vi "Read File.vi"(8 "error in (no error)":errorcluster, 10 "Parameters":refnum<class "Parameter.lvclass">[](array[class]), 11 "Parameter INI File in":refnum<class "Parameter INI File.lvclass">) -> (0 "error out":errorcluster, 2 "Parameters":refnum<class "Parameter.lvclass">[](array[class]), 3 "Parameter INI File out":refnum<class "Parameter INI File.lvclass">)   [LabVIEW 2016, in "CD Parameter Manager API.lvlib" / "Parameter INI File.lvclass"]
uses:
  Parameter INI File.lvclass
  <vilib>/Utility/config.llb/NI_LVConfig.lvlib
  <vilib>/Utility/error.llb/Error Cluster From Error Code.vi
  <vilib>/ErrorRing/Error Ring.xnode
  Boolean Parameter Class/Boolean Parameter.lvclass
  I32 Parameter Class/I32 Parameter.lvclass
  <vilib>/Utility/config.llb/Read Key (Boolean).vi
  <vilib>/Utility/config.llb/Read Key (I32).vi
  Double Parameter Class/Double Parameter.lvclass
  <vilib>/Utility/config.llb/Read Key (Double).vi
  String Parameter Class/String Parameter.lvclass
  <vilib>/Utility/config.llb/Read Key (String).vi
  Parameter Class/Parameter.lvclass
  <vilib>/Utility/config.llb/Read Key (Path).vi
  File Path Parameter Class/File Path Parameter.lvclass
  C:/Repositories/UI-Control-Initializer-API/Source/Parameter Class/Parameter.lvclass
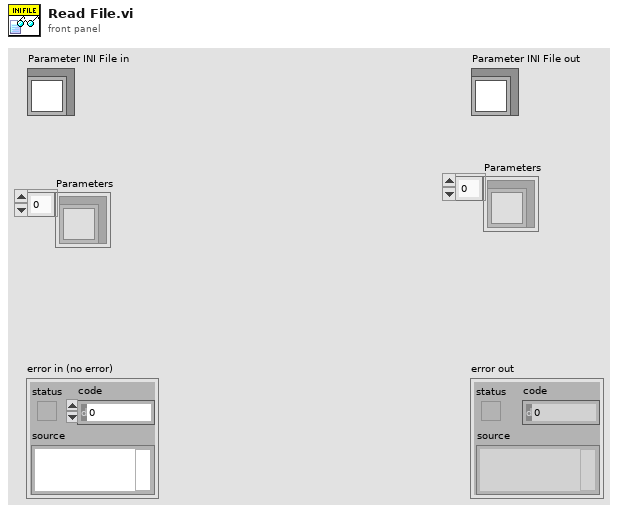
[diagram p1: front panel]
types:
  T1 = typedef "NI_LVConfig.lvlib/Config Data RefNum.ctl" = refnum<k1>
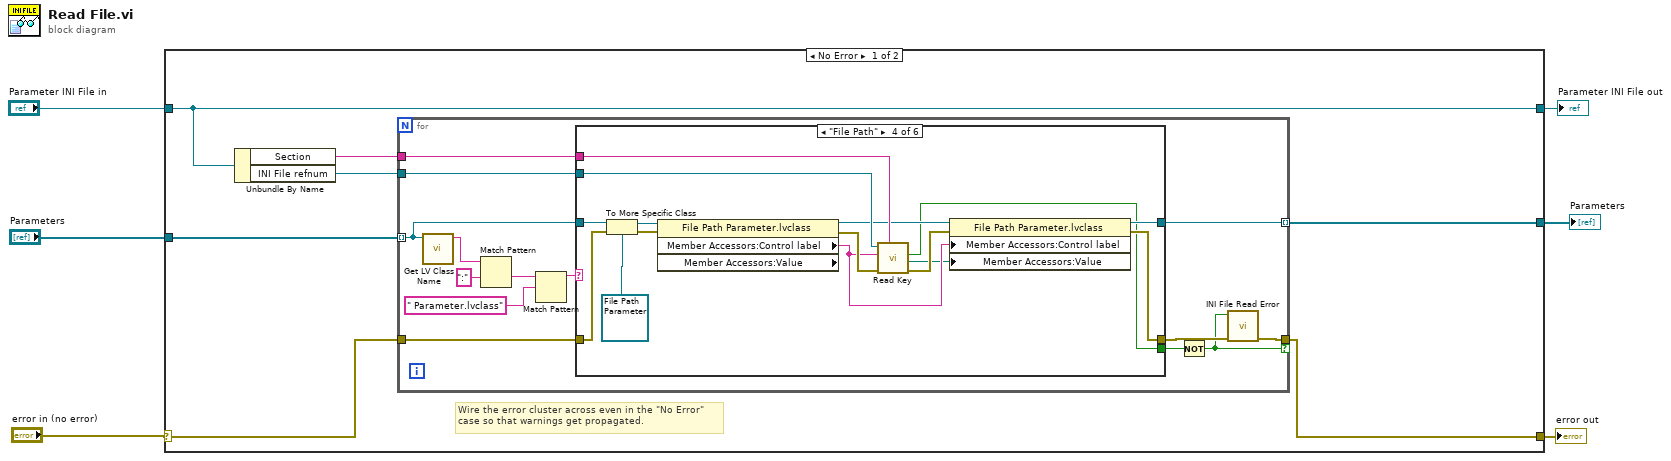
[diagram p0: block diagram]
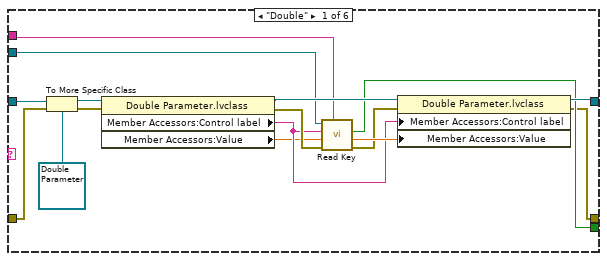
[diagram p2: hidden frame]
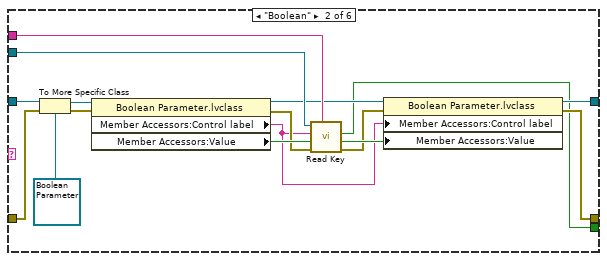
[diagram p3: hidden frame]
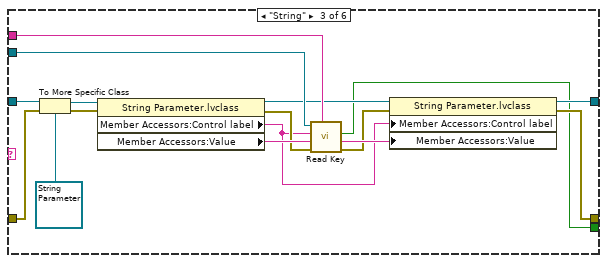
[diagram p4: hidden frame]
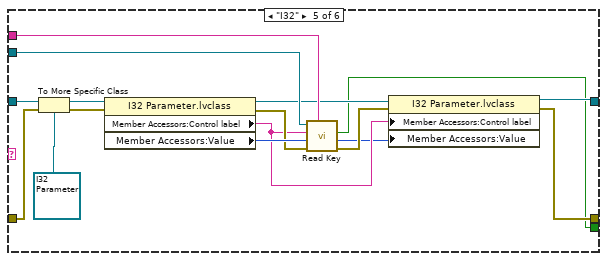
[diagram p5: hidden frame]
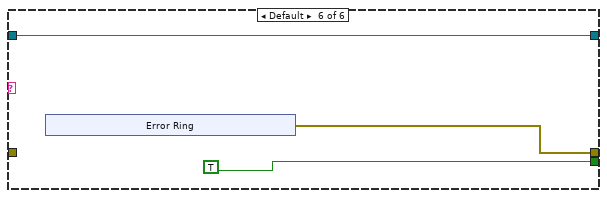
[diagram p6: hidden frame]
diagram:
  n1 = case shown="No Error" "error in (no error)" {
    selector: "error in (no error)" -> [w13 w117]
    tunnel: [w8 w117] -> w4
    tunnel: [w10 w116] -> w5
    tunnel: "Parameter INI File in" -> [w10 w116]
    tunnel: "Parameters" -> [w9 w115]
    tunnel: [w7 w115] -> w1
    frame No Error {
      # "Wire the error cluster across even in the \"No Error\"\ncase so that warnings get propagated."
      n2 = Unbundle By Name(w10) -> ("Section"=w11:string, "INI File refnum"=w12:T1)
      n3 = for {
        tunnel: w13 -> [w22]
        tunnel: [w15] -> w8 if=w14
        tunnel: w12 -> [w20]
        tunnel: w9 -> [w19] mode=indexing
        tunnel: w11 -> [w18]
        tunnel: [w17] -> w7 mode=indexing
        n4 = call <vilib>:"Get LV Class Name.vi"("object"=w19) -> ("class name"=w24:string)  [unwired: 9 in, 1 out]
        n5 = Match Pattern(string=w24, regular expression=":") -> (after substring=w26:string)  [unwired: 1 in, 3 out]
        n6 = Match Pattern(string=w26, regular expression=" Parameter.lvclass") -> (before substring=w23:string)  [unwired: 1 in, 3 out]
        n7 = case shown="\"File Path\"" w23 {
          tunnel: w22 -> [w39 w55 w71 w87 w102 _]
          tunnel: [w30 w46 w63 w80 w93 w108] -> w16
          tunnel: [w31 w44 w61 w78 w91 TRUE] -> w21
          tunnel: w20 -> [w28 w52 w68 w84 w100 _]
          tunnel: w19 -> [w42 w56 w72 w88 w103 w107]
          tunnel: w18 -> [w29 w53 w69 w85 w99 _]
          tunnel: [w32 w45 w62 w79 w96 w107] -> w17
          frame "Double" {
            n8 = To More Specific Class(target class=refnum<class "Double Parameter.lvclass"> refnum ("CD Parameter Manager API.lvlib:Double Parameter.lvclass"), reference=w42, error in=w39) -> (specific class reference=w41:refnum<class "Double Parameter.lvclass">, error out=w43:errorcluster)
            n9 = property class="Double Parameter.lvclass"(reference=w41, error in=w43) -> (reference out=w36:refnum<class "Double Parameter.lvclass">, error out=w35:errorcluster, "Member Accessors:Control label"=w34:string, "Member Accessors:Value"=w33:dbl)
            n10 = call-poly <vilib>:"Read Key.vi"("section"=w29, "error in (no error)"=w35, "default value"=w33, "key"=w34, "refnum"=w28) -> ("error out"=w37:errorcluster, "value"=w38:dbl, "found?"=w31:bool)  [unwired: 3 in, 1 out]
            n11 = property class="Double Parameter.lvclass"(reference=w36, error in=w37, "Member Accessors:Control label"=w34, "Member Accessors:Value"=w38) -> (reference out=w32:refnum<class "Double Parameter.lvclass">, error out=w30:errorcluster)
          }
          frame "Boolean" {
            n12 = To More Specific Class(target class=refnum<class "Boolean Parameter.lvclass"> refnum ("CD Parameter Manager API.lvlib:Boolean Parameter.lvclass"), reference=w56, error in=w55) -> (specific class reference=w58:refnum<class "Boolean Parameter.lvclass">, error out=w59:errorcluster)
            n13 = property class="Boolean Parameter.lvclass"(reference=w58, error in=w59) -> (reference out=w48:refnum<class "Boolean Parameter.lvclass">, error out=w54:errorcluster, "Member Accessors:Control label"=w47:string, "Member Accessors:Value"=w57:bool)
            n14 = call-poly <vilib>:"Read Key.vi"("section"=w53, "error in (no error)"=w54, "default value"=w57, "key"=w47, "refnum"=w52) -> ("error out"=w49:errorcluster, "value"=w50:bool, "found?"=w44:bool)  [unwired: 3 in, 1 out]
            n15 = property class="Boolean Parameter.lvclass"(reference=w48, error in=w49, "Member Accessors:Control label"=w47, "Member Accessors:Value"=w50) -> (reference out=w45:refnum<class "Boolean Parameter.lvclass">, error out=w46:errorcluster)
          }
          frame "String" {
            n16 = To More Specific Class(target class=refnum<class "String Parameter.lvclass"> refnum ("CD Parameter Manager API.lvlib:String Parameter.lvclass"), reference=w72, error in=w71) -> (specific class reference=w74:refnum<class "String Parameter.lvclass">, error out=w75:errorcluster)
            n17 = property class="String Parameter.lvclass"(reference=w74, error in=w75) -> (reference out=w65:refnum<class "String Parameter.lvclass">, error out=w70:errorcluster, "Member Accessors:Control label"=w64:string, "Member Accessors:Value"=w73:string)
            n18 = call-poly <vilib>:"Read Key.vi"("section"=w69, "error in (no error)"=w70, "default value"=w73, "key"=w64, "refnum"=w68) -> ("error out"=w66:errorcluster, "value"=w67:string, "found?"=w61:bool)  [unwired: 3 in, 1 out]
            n19 = property class="String Parameter.lvclass"(reference=w65, error in=w66, "Member Accessors:Control label"=w64, "Member Accessors:Value"=w67) -> (reference out=w62:refnum<class "String Parameter.lvclass">, error out=w63:errorcluster)
          }
          frame "File Path" {
            n20 = To More Specific Class(target class=refnum<class "File Path Parameter.lvclass"> refnum ("CD Parameter Manager API.lvlib:File Path Parameter.lvclass"), reference=w88, error in=w87) -> (specific class reference=w89:refnum<class "File Path Parameter.lvclass">, error out=w90:errorcluster)
            n21 = property class="File Path Parameter.lvclass" props=["Member Accessors:Control label", "Member Accessors:Value"](reference=w89, error in=w90) -> (reference out=w82:refnum<class "File Path Parameter.lvclass">, error out=w86:errorcluster, "Member Accessors:Control label"=w81:string)  [unwired: 1 out]
            n22 = call-poly <vilib>:"Read Key.vi"("section"=w85, "error in (no error)"=w86, "key"=w81, "refnum"=w84) -> ("error out"=w83:errorcluster, "value"=w76:path, "found?"=w78:bool)  [unwired: 4 in, 1 out]
            n23 = property class="File Path Parameter.lvclass"(reference=w82, error in=w83, "Member Accessors:Control label"=w81, "Member Accessors:Value"=w76) -> (reference out=w79:refnum<class "File Path Parameter.lvclass">, error out=w80:errorcluster)
          }
          frame "I32" {
            n24 = To More Specific Class(target class=refnum<class "I32 Parameter.lvclass"> refnum ("CD Parameter Manager API.lvlib:I32 Parameter.lvclass"), reference=w103, error in=w102) -> (specific class reference=w105:refnum<class "I32 Parameter.lvclass">, error out=w106:errorcluster)
            n25 = property class="I32 Parameter.lvclass"(reference=w105, error in=w106) -> (reference out=w97:refnum<class "I32 Parameter.lvclass">, error out=w101:errorcluster, "Member Accessors:Control label"=w94:string, "Member Accessors:Value"=w104:i32)
            n26 = call-poly <vilib>:"Read Key.vi"("section"=w99, "error in (no error)"=w101, "default value"=w104, "key"=w94, "refnum"=w100) -> ("error out"=w95:errorcluster, "value"=w92:i32, "found?"=w91:bool)  [unwired: 3 in, 1 out]
            n27 = property class="I32 Parameter.lvclass"(reference=w97, error in=w95, "Member Accessors:Control label"=w94, "Member Accessors:Value"=w92) -> (reference out=w96:refnum<class "I32 Parameter.lvclass">, error out=w93:errorcluster)
          }
          frame Default {
            n28 = xnode "Error Ring"() -> ("error out"=w108:errorcluster)
          }
        }
        n29 = Not(x=w21) -> (.not. x?=w14:bool)
        n30 = call "INI File Read Error.vi"("error in (no error)"=w16, "INI Key Not Found?"=w14) -> ("error out"=w15:errorcluster)  [unwired: 9 in]
      }
    }
    frame Error {
    }
  }
  "error out" <- w4
  "Parameter INI File out" <- w5
  "Parameters" <- w1
